vi "old version -- App - RUS scan V0.vi"(4 "Bypass error dialog":bool=TRUE, 5 "Divide something by something for Albert":bool=TRUE, 6 "Zero amplitude at the end":bool=TRUE, 7 "Save data settings":T3={"Save data"=TRUE, "Data Root Path"=path "C:/Data/RUS/Experiment/ProbeTest/systemtest", "File Prefix"="140.82700K_300_3300_", "File Format"=enum."BINARY", "Save column names"=TRUE, "File Comments"="<Description of the current file>", "User/Prj"="<User Name/Project Description>"}, 8 "error in (no error)":errorcluster, 9 "Fast swep settings":T1={"Update rate (Hz)"=250.0, "Start F, Hz"=300000.0, "Stop F"=1000000.0, "Number of points"=10000, "Amplitude"=2.1, "Init&amplitude"=TRUE, "IF"=1000.0, "Time constant"=0.003} {"IF" format="%#_6p"; "Amplitude" min=0.0 max=2.5; "Number of points" format="%.0p"; "Stop F" format="%#_6p"; "Start F, Hz" format="%#_6p"; "Update rate (Hz)" format="%0.2f"}, 11 "Lock-in DAQ settings":T2={"Lockin mode"=enum."NI-DAQ", "DAQmx Device"="Dev1", "SR Lockin"="GPIB0::10::INSTR", "Clock Multiplier"=64, "Low-pass filter"=enum."No filtering", "Ranges and couplings "=[{"Range"=2.5, "Coupling"=10106}], "Samples per read"=10, "Record IF"=TRUE, "Auto-phase"=TRUE} {"Ranges and couplings"."Coupling" items=["default"=-1, "RSE"=10083, "NRSE"=10078, "Differential"=10106, "Pseudodifferential"=12529]}) -> (0 "error out":errorcluster, 2 "Actual file path":path=path "C:/data/RUS/Experiment/YBCO_4/Sweep10/June_2011/061111/141.78200K_300_3300_001_061111.dat", 3 "Data":dbl[][](array[numeric]))   [LabVIEW 2012]
uses:
  RUS/Controls/Sweep settings.ctl
  File/Controls/Save data settings.ctl
  File/Controls/File formats.ctl
  <vilib>/Math Plots/2D Math Plots/2D Compass/2D Compass XCtrl/2D Compass.xctl
  <vilib>/Math Plots/2D Math Plots/2D Compass/2D Compass Datatype/2D Compass Datatype.lvclass
  RUS/Controls/Lock-in DAQ settings.ctl
  <vilib>/Utility/error.llb/DialogType.ctl
  <vilib>/Math Plots/2D Math Plots/2D Compass/2D Compass Datatype/Public/Plot Helper (Complex).vi
panel:
  in  "plot complex/IF":bool=TRUE
  out "IF":cluster{dbl[], dbl[]}[](graph)
  out "2D Compass":refnum<class "2D Plot Datatype.lvclass">[](xcontrol)
  out "Progress":u8(slide)=1 scale=0.0..100.0
  in  "Tab Control":enum32{"Main controls", "File", "Advanced"}(tab)
  in  "Manual\nPhase":dbl(slide) scale=-180.0..180.0
  out "Error status byte\n(bit 5 - FAST aborted)":u8 format="%08b"
  out "STD status byte":u8 format="%08b"
  out "DO array  making time":u32=151
  out "DO write time, ms":u32=611162
  out "Loop counter":i32=15000
  in  "Graph update rate, ms":u32=100
  in  "Plot when running":bool=TRUE
  out "Pre-sweep delay, s":dbl=15.2
  out "Samples in buffer":u32
  out "Actual setup time, ms":u32=1504
  out "SpaceAvail":u32=4967
  in  "stop":bool
  out "XY Graph":cluster{dbl[], dbl[]}[](graph)
  # "SRS Lockin related"
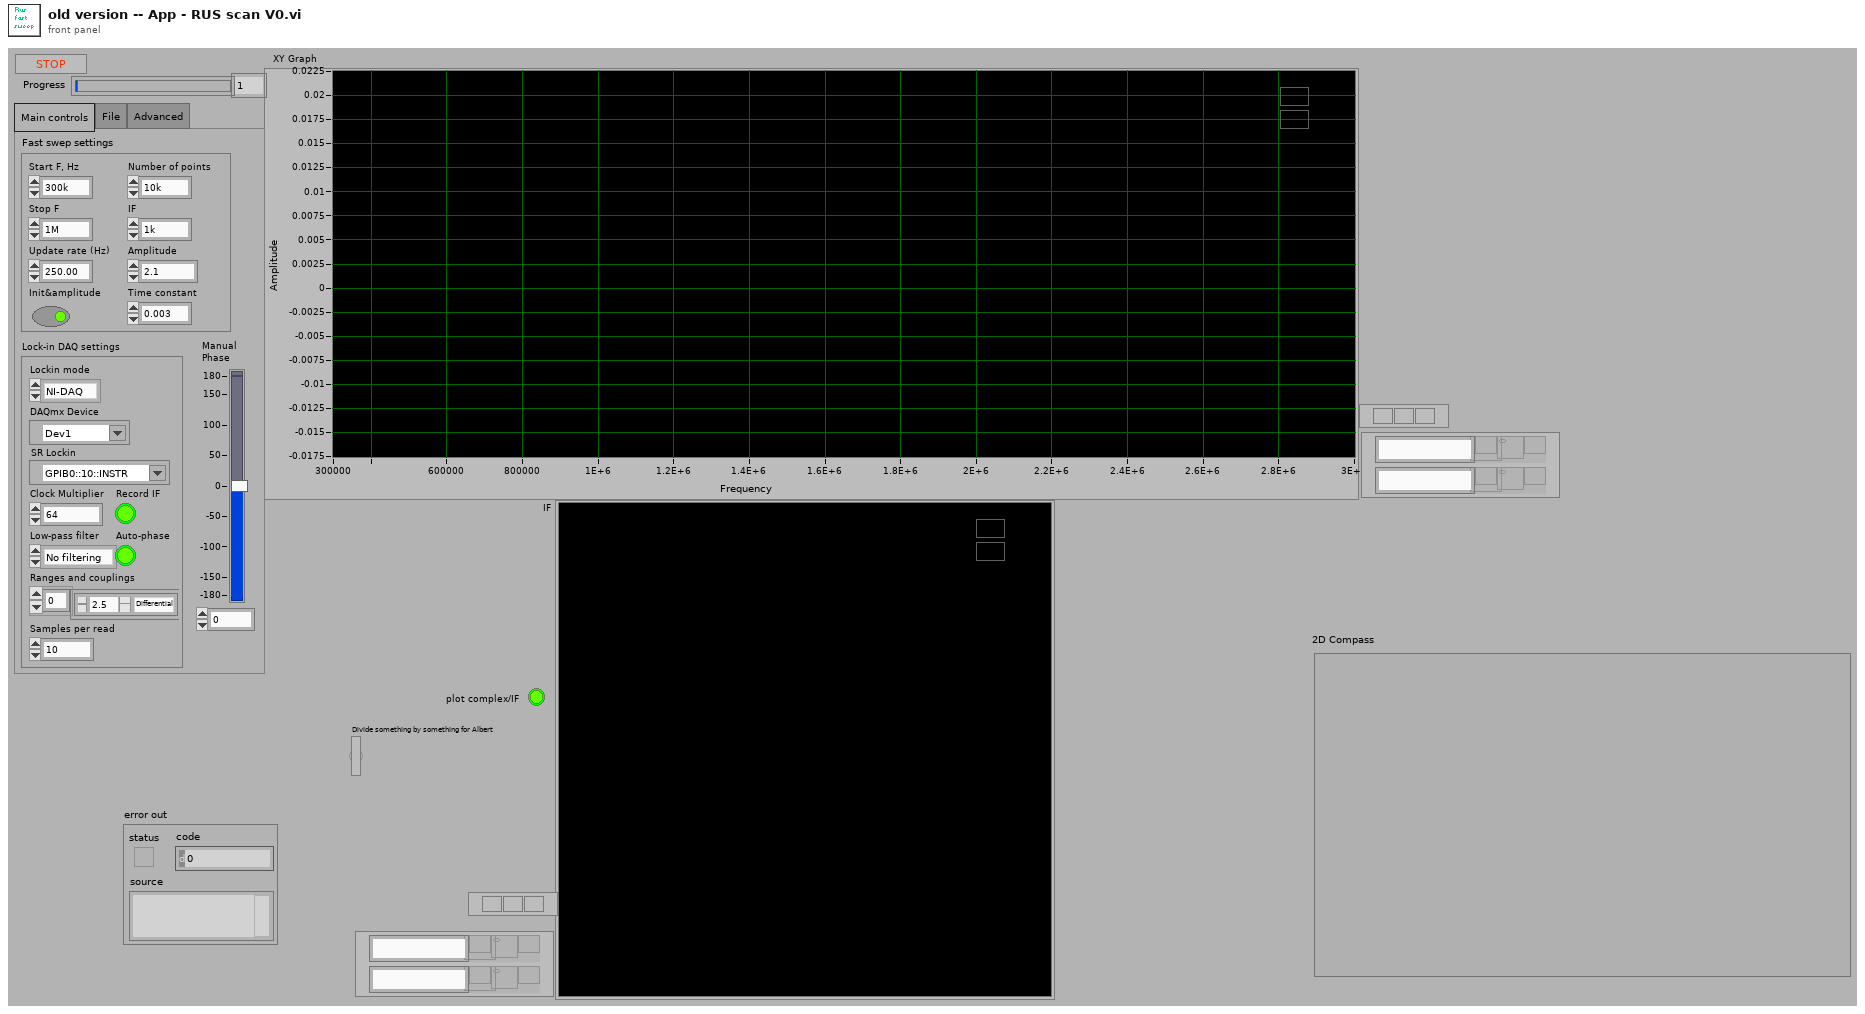
[diagram p1: front panel]
types:
  T1 = typedef "Sweep settings.ctl" = cluster{"Update rate (Hz)":dbl, "Start F, Hz":dbl, "Stop F":dbl, "Number of points":i32, "Amplitude":dbl, "Init&amplitude":bool, "IF":dbl, "Time constant":dbl}
  T2 = typedef "Lock-in DAQ settings.ctl" = cluster{"Lockin mode":enum16{"SRS", "NI-DAQ"}, "DAQmx Device":tag, "SR Lockin":refnum<visa-resource-name>, "Clock Multiplier":i32, "Low-pass filter":enum16{"No filtering", "Butterworth", "Bessel"}, "Ranges and couplings ":cluster{"Range":dbl, "Coupling":i32}[], "Samples per read":i32, "Record IF":bool, "Auto-phase":bool}
  T3 = typedef "Save data settings.ctl" = cluster{"Save data":bool, "Data Root Path":path, "File Prefix":string, "File Format":T4, "Save column names":bool, "File Comments":string, "User/Prj":string}
  T4 = typedef "File formats.ctl" = enum16{"TDMS", "ASCII", "BINARY"}
  T5 = typedef "RUS settings.ctl" = cluster{"NI-DAQ lockin settings":T6, "Fast swep settings":T1, "Pre-sweep delay, s":dbl, "Lockin mode":enum16{"SRS", "NI-DAQ"}, "SR Lockin":refnum<visa-resource-name>, "DAQmx Device":tag, "Clock Multiplier":i32, "Fast Sweep Data Out":cluster{"DO clock task":refnum<k21>, "DO task":refnum<k21>, "Update clock task":refnum<k21>, "DAQ lockin task":refnum<k21>, "Pre-sweep counter task":refnum<k21>}, "Lockin Range, V":sgl, "F Array":dbl[], "Freq. update clock terminal":string, "DO Clock Rate (Hz)":dbl, "ADC clock terminal":string, "Pre-sweep counter terminal":string, "Samples per read":i32, "DO clock terminal":string, "Pre-sweep points":i32, "F points per write":i32, "Total sweep time, s":dbl, "Initial SYNTH phase":dbl, "Record IF":bool, "Save data settings":T3, "Data file path":path, "New data user event":refnum<user-event>, "Stop user event":refnum<user-event>, "Number of channels":i32, "Auto-phase":bool}
  T6 = typedef "RUS NI-DAQ Lockin Settings.ctl" = cluster{"Samples per sine wave":i32, "Sine waves per freq step":i32, "Output Representation":enum16{"Real/Imaginary", "Polar"}, "Low-pass filter":enum16{"No filtering", "Butterworth", "Bessel"}, "Ranges and couplings ":cluster{"Range":dbl, "Coupling":i32}[]}
  T7 = typedef "DialogType.ctl" = u16
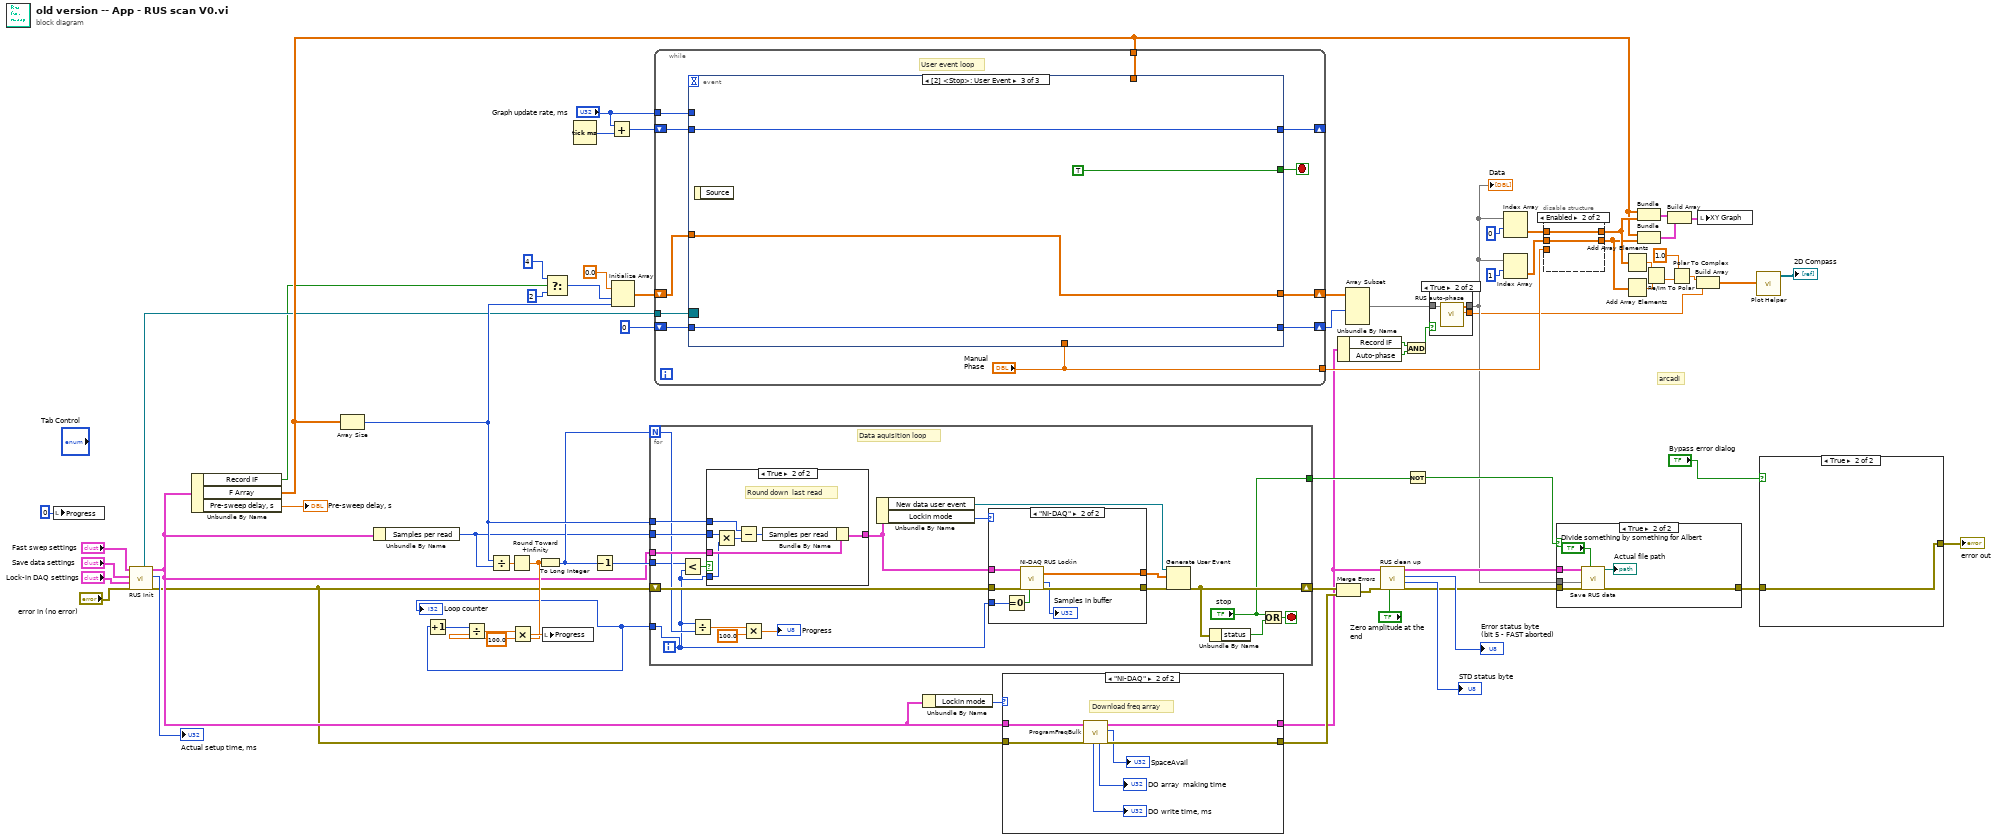
[diagram p0: block diagram]
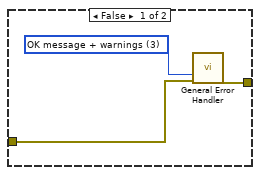
[diagram p2: hidden frame]
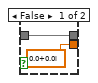
[diagram p3: hidden frame]
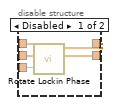
[diagram p5: hidden frame]
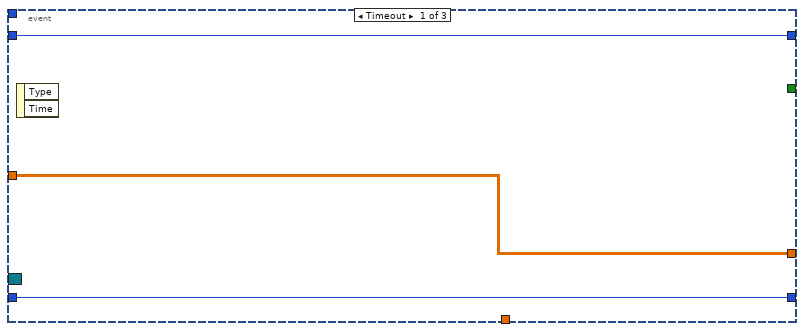
[diagram p6: hidden frame]
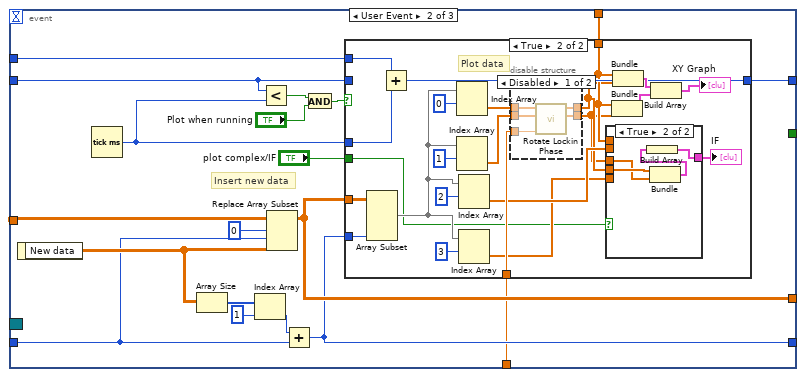
[diagram p7: hidden frame]
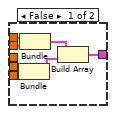
[diagram p9: hidden frame]
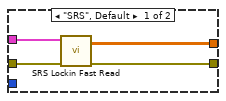
[diagram p13: hidden frame]
diagram:
  # "arcadi"
  n1 = local write "Progress"(u8 0 ("Progress")) -> ()
  n2 = call "RUS Init.vi"("error in (no error)"="error in (no error)", "Lock-in DAQ settings"="Lock-in DAQ settings", "Save data settings"="Save data settings", "Fast swep settings"="Fast swep settings") -> ("error out"=w23:errorcluster, "Actual setup time, ms"=→"Actual setup time, ms":u32, "RUS settings out"=w24:T5, "Event Registration Refnum"=w18:refnum<event-registration>)  [unwired: 4 in]
  n3 = Unbundle By Name(w24) -> ("Record IF"=w11:bool, "F Array"=w19:dbl[], "Pre-sweep delay, s"=→"Pre-sweep delay, s":dbl)
  n4 = Array Size(array=w19) -> (size(s)=w38:i32)
  n5 = Unbundle By Name(w24) -> ("Samples per read"=w30:i32)
  n6 = Divide(x=w38, y=w30) -> (x/y=w70:dbl)
  n7 = Round Toward +Infinity(x=w70) -> (ceil(x): smallest int >= x=w64:dbl)
  n8 = To Long Integer(number=w64) -> (32bit integer=w31:i32)
  n9 = Select(t=4 ("dimension size"), s=w11, f=2 ("dimension size")) -> (s? t:f=w14:i32)
  n10 = Tick Count (ms)() -> (millisecond timer value=w71:u32)
  n11 = Decrement(x=w31) -> (x-1=w60:i32)
  n12 = Add(x="Graph update rate, ms", y=w71) -> (x+y=w21:u32)
  n13 = Initialize Array(0.0 ("Numeric"), w14, w38) -> (w62:dbl[][])
  n14 = for {
    N: w31 -> [w81]
    shift-right: [w89] -> w34
    shift-left: w23 -> [w92]
    tunnel: w30 -> [w85]
    tunnel: [w76] -> w63
    tunnel: w60 -> [w77]
    tunnel: w38 -> [w86]
    tunnel: w24 -> [w84]
    tunnel: ["stop"] -> w50
    i -> [w76]
    stop <- w91 stop-if-true
    # "Data aquisition loop"
    n15 = Less?(x=w77, y=w76) -> (x < y?=w87:bool)
    n16 = Divide(x=w76, y=w81) -> (x/y=w80:dbl)
    n17 = case shown="True" w87 {
      tunnel: w86 -> [_ w100]
      tunnel: w85 -> [_ w95]
      tunnel: w76 -> [_ w94]
      tunnel: w84 -> [w93 w98]
      tunnel: [w93 w96] -> w83
      frame False {
      }
      frame True {
        # "Round down  last read"
        n18 = Multiply(x=w95, y=w94) -> (x*y=w99:i32)
        n19 = Subtract(x=w100, y=w99) -> (x-y=w97:i32)
        n20 = Bundle By Name(cluster=w98, "Samples per read"=w97) -> (w96:T5)
      }
    }
    n21 = Multiply(x=w80, y=100.0) -> (x*y=→"Progress":dbl)
    n22 = Unbundle By Name(w83) -> ("New data user event"=w73:refnum<user-event>, "Lockin mode"=w82:enum16{"SRS", "NI-DAQ"})
    n23 = case shown="\"NI-DAQ\"" w82 {
      tunnel: w92 -> [w104 w111]
      tunnel: [w103 w110] -> w90
      tunnel: [w102 w109] -> w88
      tunnel: w83 -> [w101 w108]
      tunnel: w76 -> [_ w105]
      frame "SRS", Default {
        n24 = call "SRS Lockin Fast Read.vi"("error in (no error)"=w104, "RUS settings"=w101) -> ("error out"=w103:errorcluster, "Lockin out"=w102:dbl[][])  [unwired: 4 in, 4 out]
      }
      frame "NI-DAQ" {
        n25 = Equal To 0?(x=w105) -> (x = 0?=w106:bool)
        n26 = call "NI-DAQ RUS Lockin.vi"("Init?"=w106, "error in (no error)"=w111, "RUS settings"=w108) -> ("error out"=w110:errorcluster, "AvailSampPerChan"=→"Samples in buffer":u32, "Lockin out"=w109:dbl[][])  [unwired: 5 in, 1 out]
      }
    }
    n27 = Generate User Event(user event=w73, event data cluster=w88, error in=w90) -> (error out=w89:errorcluster)  [unwired: 1 out]
    n28 = Unbundle By Name(w89) -> ("status"=w74:bool)
    n29 = Or(x="stop", y=w74) -> (x .or. y?=w91:bool)
  }
  "Loop counter" <- w63
  n30 = Increment(x=w63) -> (x+1=w59:i32)
  n31 = Divide(x=w59, y=w64) -> (x/y=w67:dbl)
  n32 = Multiply(x=w67, y=100.0) -> (x*y=w65:dbl)
  n33 = local write "Progress"(w65) -> ()
  n34 = while {
    tunnel: w18 -> [w122]
    shift-right: [w120] -> w52
    shift-left: w62 -> [w119]
    shift-right: [w116] -> _
    shift-left: w21 -> [w118]
    tunnel: "Graph update rate, ms" -> [w117]
    shift-right: [w114] -> w51
    shift-left: 0 ("disabled index (col)") -> [w115]
    tunnel: w19 -> [w113]
    tunnel: ["Manual\nPhase"] -> w48
    stop <- w121 stop-if-true
    # "User event loop"
    n35 = event shown="[2] <Stop>: User Event" {
      selector: w122 -> [_ _ _]
      dyn-events: _ -> [_ _ _]
      timeout: _ -> [_ _ _]
      tunnel: [_ _ TRUE] -> w121
      tunnel: [w125 w138 w188] -> w120
      tunnel: w119 -> [w125 w142 w188]
      tunnel: w118 -> [w124 w129 w187]
      tunnel: w117 -> [_ w127 _]
      tunnel: [w124 w144 w187] -> w116
      tunnel: w115 -> [w123 w130 w186]
      tunnel: [w123 w136 w186] -> w114
      tunnel: w113 -> [_ w137 _]
      tunnel: "Manual\nPhase" -> [_ w135 _]
      event Timeout {
        n36 = event-data() -> ()  [unwired: 3 out]
      }
      event User Event {
        # "Insert new data"
        n37 = event-data() -> ("New data"=w141:dbl[][])  [unwired: 1 out]
        n38 = Tick Count (ms)() -> (millisecond timer value=w128:u32)
        n39 = Array Size(array=w141) -> (size(s)=w140:i32[])
        n40 = Index Array(array=w140, index=1) -> (element=w131:i32)
        n41 = Less?(x=w129, y=w128) -> (x < y?=w133:bool)
        n42 = Replace Array Subset(array=w142, new element=w141, index (row)=0 ("disabled index (col)"), index (col)=w130) -> (w138:dbl[][])
        n43 = Add(x=w131, y=w130) -> (x+y=w136:i32)
        n44 = And(x=w133, y="Plot when running") -> (x .and. y?=w143:bool)
        n45 = case shown="True" w143 {
          tunnel: w138 -> [_ w164]
          tunnel: w128 -> [_ w157]
          tunnel: [w145 w156] -> w144
          tunnel: w129 -> [w145 _]
          tunnel: w137 -> [_ w155]
          tunnel: w136 -> [_ w159]
          tunnel: w135 -> [_ w162]
          tunnel: w127 -> [_ w158]
          tunnel: "plot complex/IF" -> [_ w148]
          frame False {
          }
          frame True {
            # "Plot data"
            n46 = Array Subset(array=w164, length (col)=w159) -> (w152:dbl[][])  [unwired: 3 in]
            n47 = Add(x=w158, y=w157) -> (x+y=w156:u32)
            n48 = Index Array(array=w152, index (row)=0) -> (element=w167:dbl[])  [unwired: 1 in]
            n49 = Index Array(array=w152, index (row)=1) -> (element=w168:dbl[])  [unwired: 1 in]
            n50 = Index Array(array=w152, index (row)=2) -> (element=w151:dbl[])  [unwired: 1 in]
            n51 = Index Array(array=w152, index (row)=3) -> (element=w150:dbl[])  [unwired: 1 in]
            n52 = disable-structure shown="Disabled" {
              disable-tunnel: w168 -> [w183 w184]
              disable-tunnel: w167 -> [w182 w185]
              disable-tunnel: [w181 w185] -> w147
              disable-tunnel: [w180 w184] -> w146
              disable-tunnel: w162 -> [w179 _]
              frame Disabled {
                n53 = call "Rotate Lockin Phase.vi"("Phase"=w179, "Array Y in"=w183, "Array X in"=w182) -> ("Array Y out"=w180:dbl[], "Array X out"=w181:dbl[])  [unwired: 7 out]
              }
              frame Enabled {
              }
            }
            n54 = case shown="True" w148 {
              tunnel: w155 -> [w174 _]
              tunnel: w151 -> [w173 _]
              tunnel: w150 -> [w172 _]
              tunnel: [w169 w175] -> w149
              tunnel: w147 -> [_ w178]
              tunnel: w146 -> [_ w177]
              frame False {
                n55 = Bundle("F Array"=w174, w172) -> (w170:cluster{"F Array":dbl[], dbl[]})  [unwired: 1 out]
                n56 = Bundle("F Array"=w174, w173) -> (w171:cluster{"F Array":dbl[], dbl[]})  [unwired: 1 out]
                n57 = Build Array(w171, w170) -> (w169:cluster{"F Array":dbl[], dbl[]}[])
              }
              frame True {
                n58 = Bundle(w178, w177) -> (w176:cluster{dbl[], dbl[]})  [unwired: 1 out]
                n59 = Build Array(w176) -> (w175:cluster{dbl[], dbl[]}[])
              }
            }
            "IF" <- w149
            n60 = Bundle("F Array"=w155, w146) -> (w163:cluster{"F Array":dbl[], dbl[]})  [unwired: 1 out]
            n61 = Bundle("F Array"=w155, w147) -> (w166:cluster{"F Array":dbl[], dbl[]})  [unwired: 1 out]
            n62 = Build Array(w166, w163) -> (→"XY Graph":cluster{"F Array":dbl[], dbl[]}[])
          }
        }
      }
      event User Event {
        n63 = event-data() -> ()  [unwired: 2 out]
      }
    }
  }
  n64 = Unbundle By Name(w24) -> ("Lockin mode"=w46:enum16{"SRS", "NI-DAQ"})
  n65 = case shown="\"NI-DAQ\"" w46 {
    tunnel: w24 -> [w190 w198]
    tunnel: w23 -> [w191 w197]
    tunnel: [w191 w196] -> w47
    tunnel: [w190 w192] -> w10
    frame "SRS", Default {
    }
    frame "NI-DAQ" {
      # "Download freq array"
      n66 = call "ProgramFreqBulk.vi"("error in (no error)"=w197, "RUS settings"=w198) -> ("error out"=w196:errorcluster, "SpaceAvail"=→"SpaceAvail":u32, "RUS settings out"=w192:T5, "DO array  making time"=→"DO array  making time":u32, "DO write time"=→"DO write time, ms":u32)  [unwired: 3 in, 2 out]
    }
  }
  n67 = Merge Errors(w34, w47) -> (w33:errorcluster)
  n68 = Unbundle By Name(w10) -> ("Record IF"=w9:bool, "Auto-phase"=w8:bool)
  n69 = Array Subset(array=w52, length (row)=w51) -> (w6:dbl[][])  [unwired: 3 in]
  n70 = call "RUS clean up.vi"("Zero amplitude at the end"="Zero amplitude at the end", "error in (no error)"=w33, "RUS settings"=w10) -> ("error out"=w32:errorcluster, "STD status byte"=→"STD status byte":u8, "Error status byte\n(bit 5 - FAST aborted)"=→"Error status byte\n(bit 5 - FAST aborted)":u8, "RUS settings out"=w26:T5)  [unwired: 5 in]
  n71 = And(x=w9, y=w8) -> (x .and. y?=w7:bool)
  n72 = Not(x=w50) -> (.not. x?=w22:bool)
  n73 = case shown="True" w7 {
    tunnel: w6 -> [w200 w203]
    tunnel: [w200 w202] -> w5
    tunnel: [cdb 0.0+0.0i ("Reference") w201] -> w4
    frame False {
    }
    frame True {
      n74 = call "RUS auto-phase.vi"("Data in"=w203) -> ("Reference"=w201:cdb, "Data out"=w202:dbl[][])  [unwired: 9 in]
    }
  }
  "Data" <- w5
  n75 = Index Array(array=w5, index (row)=0) -> (element=w57:dbl[])  [unwired: 1 in]
  n76 = Index Array(array=w5, index (row)=1) -> (element=w58:dbl[])  [unwired: 1 in]
  n77 = disable-structure shown="Enabled" {
    disable-tunnel: w58 -> [w208 w210]
    disable-tunnel: w57 -> [w207 w209]
    disable-tunnel: [w206 w209] -> w41
    disable-tunnel: [w205 w210] -> w39
    disable-tunnel: w48 -> [w204 _]
    frame Disabled {
      n78 = call "Rotate Lockin Phase.vi"("Phase"=w204, "Array Y in"=w208, "Array X in"=w207) -> ("Array Y out"=w205:dbl[], "Array X out"=w206:dbl[])  [unwired: 7 out]
    }
    frame Enabled {
    }
  }
  n79 = case shown="True" w22 {
    tunnel: w32 -> [w211 w217]
    tunnel: [w211 w215] -> w69
    tunnel: w5 -> [_ w214]
    tunnel: w26 -> [_ w213]
    frame False {
    }
    frame True {
      n80 = call "Save RUS data.vi"("Divide something by something for Albert"="Divide something by something for Albert", "error in (no error)"=w217, "Signal"=w214, "RUS settings"=w213) -> ("error out"=w215:errorcluster, "Actual file path"=→"Actual file path":path)  [unwired: 6 in]
    }
  }
  n81 = Add Array Elements(numeric array=w41) -> (sum=w44:dbl)
  n82 = Add Array Elements(numeric array=w39) -> (sum=w43:dbl)
  n83 = Bundle("F Array"=w19, "Data out"=w41) -> (w56:cluster{"F Array":dbl[], "Data out":dbl[]})  [unwired: 1 out]
  n84 = Bundle("F Array"=w19, "Data out"=w39) -> (w55:cluster{"F Array":dbl[], "Data out":dbl[]})  [unwired: 1 out]
  n85 = Re/Im To Polar(2:w43, 3:w44) -> (0:w3:dbl)  [unwired: 1 out]
  n86 = Build Array(w56, w55) -> (w54:cluster{"F Array":dbl[], "Data out":dbl[]}[])
  n87 = Polar To Complex(1:w3, 2:1.0 ("r")) -> (0:w40:cdb)
  n88 = Build Array(w40, w4) -> (w42:cdb[])
  n89 = local write "XY Graph"(w54) -> ()
  n90 = call-poly <vilib>:"Plot Helper.vi"("z vector"=w42) -> ("2D Plot Class Obj Array out"=→"2D Compass":refnum<class "2D Plot Datatype.lvclass">[])  [unwired: 2 in, 8 out]
  n91 = case shown="True" "Bypass error dialog" {
    tunnel: [w219 w221] -> w72
    tunnel: w69 -> [w218 w221]
    frame False {
      w220 = T7 3 items=["no dialog", "OK message", "continue or stop message", "OK message + warnings", "continue/stop + warnings"] ("type of dialog (OK msg:1)")
      n92 = call <vilib>:"General Error Handler.vi"("type of dialog (OK msg:1)"=w220, "error in (no error)"=w218) -> ("error out"=w219:errorcluster)  [unwired: 13 out]
    }
    frame True {
    }
  }
  "error out" <- w72
